vi "o.vi"() -> ()   [LabVIEW 2017]
panel:
  in  "Multicolumn Listbox 2":i32(listbox)
  in  "WebBrowser 2":refnum<k7>(container)
  out "element 2":string
  in  "stop":bool
  in  "y":i64=50
  out "Array":i64[](array[numeric])
  in  "Path":path
  out "e":path[](array[path])
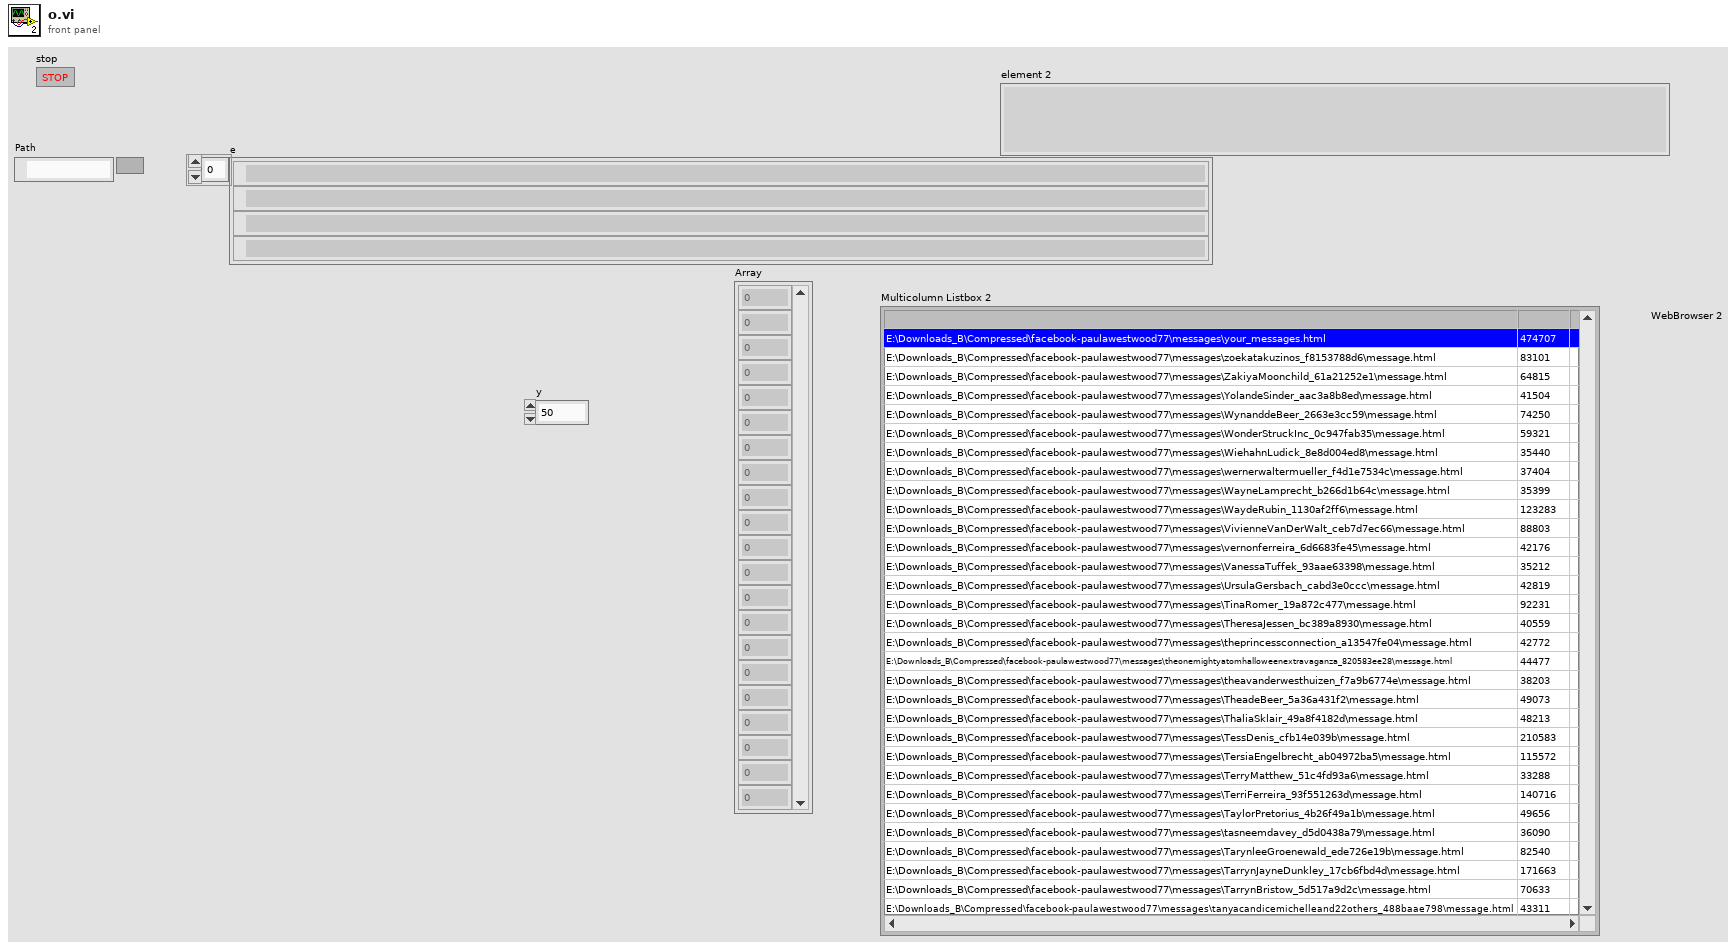
[diagram p1: front panel]
types:
  T1 = enum32{"No PSP", "Read", "Write", "Write & Read"}
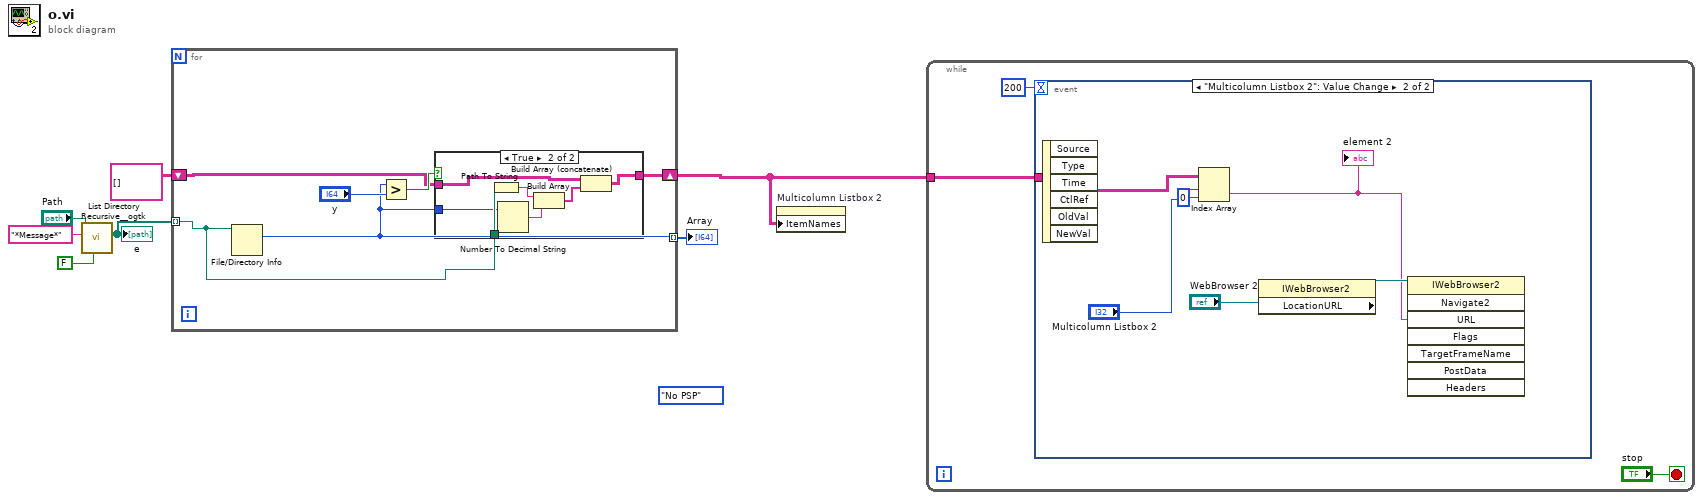
[diagram p0: block diagram]
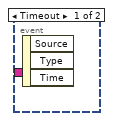
[diagram p2: hidden frame]
diagram:
  (unwired) T1."No PSP" ("Mode")
  n1 = call <userlib>:"List Directory Recursive__ogtk.vi"("List only Top-Level files in llbs? (FALSE)"=FALSE, "pattern"="*Message*", "Path"="Path") -> ("file paths"=w4:path[])  [unwired: 5 in, 3 out]
  "e" <- w4
  n2 = for {
    tunnel: w4 -> [w11] mode=indexing
    tunnel: [w8] -> w3 mode=indexing
    shift-right: [w10] -> w2
    shift-left: string[][] [] -> [w9]
    n3 = File/Directory Info(path=w11) -> (size=w8:i64)  [unwired: 1 in, 6 out]
    n4 = Greater?(x=w8, y="y") -> (0:w12:bool)
    n5 = case shown="True" w12 {
      tunnel: w11 -> [_ w20]
      tunnel: [w14 w21] -> w10
      tunnel: w9 -> [w14 w19]
      tunnel: w8 -> [_ w16]
      frame False {
      }
      frame True {
        n6 = Path To String(path=w20) -> (string=w18:string)
        n7 = Number To Decimal String(number=w16) -> (decimal integer string=w17:string)  [unwired: 1 in]
        n8 = Build Array(w18, w17) -> (w15:string[])
        n9 = Build Array (concatenate)(w19, w15) -> (w21:string[][])
      }
    }
  }
  "Array" <- w3
  n10 = property on="Multicolumn Listbox 2" class="MCListbox (strict)"("ItemNames"=w2) -> ()  [unwired: 2 in, 2 out]
  n11 = while {
    tunnel: w2 -> [w24]
    stop <- "stop" stop-if-true
    n12 = event shown="[1] \"Multicolumn Listbox 2\": Value Change" {
      selector: _ -> [_ _]
      dyn-events: _ -> [_ _]
      timeout: 200 -> [_ _]
      tunnel: w24 -> [_ w30]
      event Timeout {
        n13 = event-data() -> ()  [unwired: 1 in, 3 out]
      }
      event "Multicolumn Listbox 2": Value Change {
        n14 = event-data() -> ()  [unwired: 1 in, 6 out]
        n15 = Index Array(array=w30, index (row)="Multicolumn Listbox 2", index (col)=0 ("disabled index (col)")) -> (element=w25:string)
        "element 2" <- w25
        n16 = property class="IWebBrowser2" props=["LocationURL"](reference="WebBrowser 2") -> (reference out=w26:refnum<k7>)  [unwired: 1 in, 2 out]
        n17 = invoke class="IWebBrowser2" method="Navigate2"(reference=w26, "URL"=w25) -> ()  [unwired: 6 in, 8 out]
      }
    }
  }
